vi "Launch Async.vi"(8 "error in (no error)":errorcluster, 11 "Module in":refnum<class "Module.lvclass">) -> (0 "error out":errorcluster, 2 "MessageQ":refnum<class "MessageQ.lvclass">)   [LabVIEW 2020, in "Volatus.lvlib" / "Module.lvclass"]
uses:
  Module.lvclass
  MessageQ/MessageQ.lvclass
  MessageQ Value/MessageQ Value.lvclass
  C:/dev/lv20CE/relink/lv-promises/Promises/Value/Value.lvclass
  lv-promises/Promises/Promise/Promise.lvclass/Promise.ctl
  lv-promises/Promises/Future/Future.lvclass/Future.ctl
  MessageQ Value/MessageQ Value.lvclass/MessageQ Value.ctl
  Async Core.vi
  lv-promises/Promises/Future/Future.lvclass
  lv-promises/Promises/Promise/Promise.lvclass
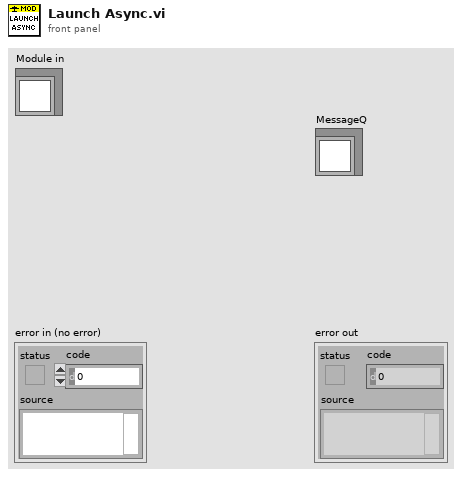
[diagram p1: front panel]
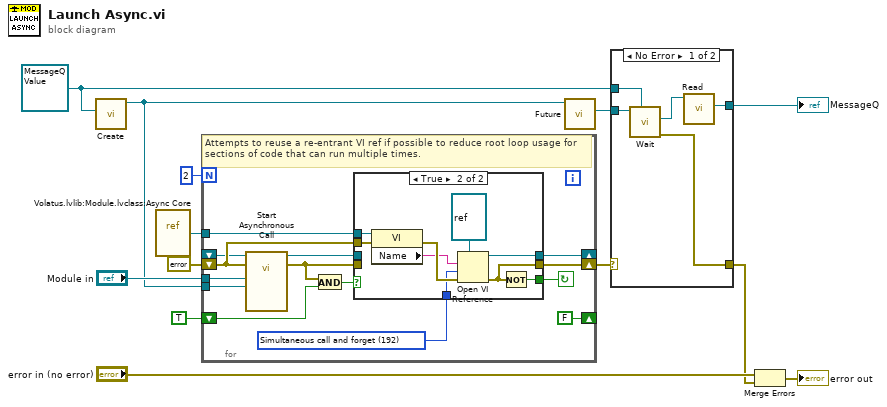
[diagram p0: block diagram]
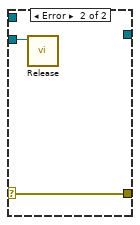
[diagram p2: hidden frame]
diagram:
  w4 = refnum<class "MessageQ Value.lvclass"> refnum ("Volatus:MessageQ Value.lvclass")
  n1 = call "Create.vi"("Result Type"=w4) -> ("Promise"=w7:refnum<class "Promise.lvclass">)  [unwired: 9 in, 1 out]
  n2 = vi-ref "Volatus.lvlib:Module.lvclass:Async Core.vi"() -> (w10:refnum<vi>)
  n3 = for {
    N: 2 -> [_]
    tunnel: w10 -> [w26]
    shift-right: [w25] -> _
    shift-left: _ -> [w24]
    shift-right: [w22] -> w6
    shift-left: errorcluster {"status"=FALSE, "code"=0, "source"=""} ("error constant") -> [w27]
    shift-right: [FALSE] -> _
    shift-left: TRUE -> [w19]
    tunnel: w7 -> [w15]
    tunnel: "Module in" -> [w14]
    stop <- w18 continue-if-true
    w16 = 192 items=["Record modifications"=1, "Open templates for editing"=2, "Prompt user to save"=4, "Prepare for reentrant run"=8, "Prompt to find missing subVIs"=16, "Hide loading dialog box"=32, "Enable simultaneous calls"=64, "Prepare to call and forget"=128, "Simultaneous call and forget"=192, "Prepare to call and collect"=256, "Simultaneous call and collect"=320]
    # "Attempts to reuse a re-entrant VI ref if possible to reduce root loop usage for sections of code that can run multiple times."
    n4 = call-by-ref "Start Asynchronous Call"(reference=w24, error in=w27, "Startup Promise"=w15, "Module in"=w14) -> (reference out=w23:refnum<vi>, error out=w21:errorcluster)  [unwired: 10 in]
    n5 = And(x=w21, y=w19) -> (x .and. y?=w20:bool)
    n6 = case shown="True" w20 {
      tunnel: w26 -> [_ w37]
      tunnel: w16 -> [_ w35]
      tunnel: [w29 w34] -> w25
      tunnel: w23 -> [w29 _]
      tunnel: [w28 w32] -> w22
      tunnel: w21 -> [w28 _]
      tunnel: w27 -> [_ w33]
      tunnel: [_ w31] -> w18
      frame False {
      }
      frame True {
        n7 = property class="VI"(reference=w37, error in=w33) -> (error out=w38:errorcluster, "Name"=w36:string)  [unwired: 1 out]
        n8 = Open VI Reference(type specifier VI Refnum (for type only)=refnum<vi> refnum, vi path=w36, options=w35, error in (no error)=w38) -> (vi reference=w34:refnum<vi>, error out=w32:errorcluster)  [unwired: 2 in]
        n9 = Not(x=w32) -> (.not. x?=w31:bool)
      }
    }
  }
  n10 = call "Future.vi"("Promise in"=w7) -> ("Future"=w5:refnum<class "Future.lvclass">)  [unwired: 9 in, 1 out]
  n11 = case shown="No Error" w6 {
    selector: w6 -> [_ w44]
    tunnel: w5 -> [w43 w45]
    tunnel: [w41 w44] -> w2
    tunnel: w4 -> [w42 _]
    tunnel: [w39 _] -> w1
    frame No Error {
      n12 = call "Wait.vi"("Result Type"=w42, "Future in"=w43) -> ("error out"=w41:errorcluster, "Result"=w40:refnum<class "MessageQ Value.lvclass">)  [unwired: 8 in]
      n13 = call "Read.vi"("MessageQ Value in"=w40) -> ("MessageQ"=w39:refnum<class "MessageQ.lvclass">)  [unwired: 10 in]
    }
    frame Error {
      n14 = call "Release.vi"("Future in"=w45) -> ()  [unwired: 11 in]
    }
  }
  "MessageQ" <- w1
  n15 = Merge Errors("error in (no error)", w2) -> (→"error out":errorcluster)
